vi "Abrir Archivo.vi"(11 "MulticolumnListbox in":refnum<vi>) -> (3 "Byte Stream File out":refnum<file>)   [LabVIEW 2020]
uses:
  <vilib>/Utility/miscctls.llb/LVRowAndColumnUnsignedTypeDef.ctl
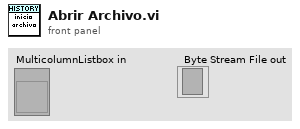
[diagram p1: front panel]
types:
  T1 = enum16{"open", "replace", "create", "open or create", "replace or create", "replace or create with confirmation"}
  T2 = typedef "LVRowAndColumnUnsignedTypeDef.ctl" = cluster{"Row":u32, "Column":u32}
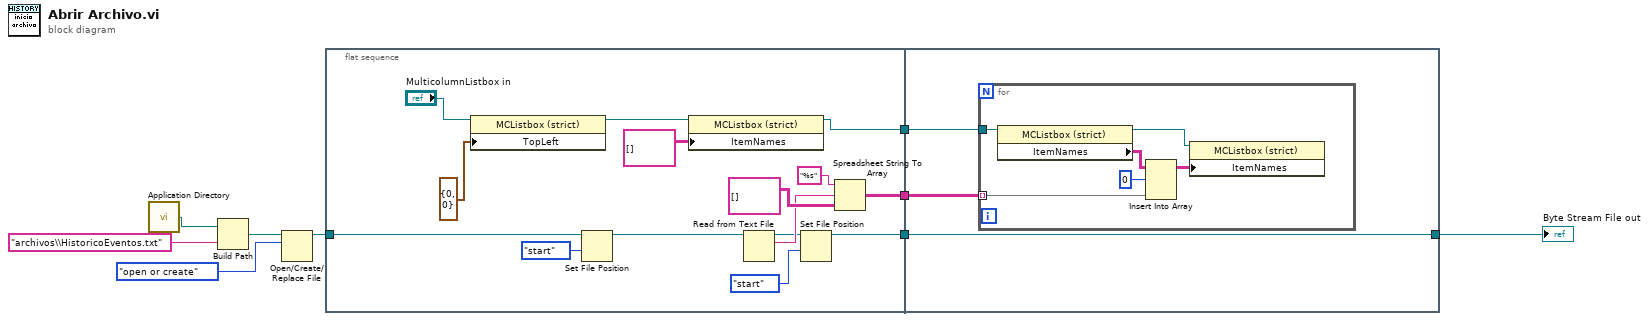
[diagram p0: block diagram]
diagram:
  n1 = call <vilib>:"Application Directory.vi"() -> ("Application Directory"=w2:path)
  n2 = Build Path(base path=w2, name or relative path="archivos\\HistoricoEventos.txt") -> (appended path=w4:path)
  n3 = Open/Create/Replace File(file path (use dialog)=w4, operation (0:open)=T1."open or create") -> (refnum out=w6:refnum<file>)  [unwired: 4 in, 2 out]
  n4 = flat-sequence {
    tunnel: w6 -> [w16]
    tunnel: [w20] -> w9
    tunnel: [w14] -> w8
    tunnel: [w13] -> w7
    tunnel: w9 -> [w27]
    tunnel: [w26] -> w1
    tunnel: w8 -> [w26]
    tunnel: w7 -> [w25]
    frame #0 {
      n5 = property on="Property Node" class="MCListbox (strict)"(reference="MulticolumnListbox in", "TopLeft"=T2 {"Row"=0, "Column"=0} ("Top Left Visible Cell")) -> (reference out=w10:refnum<vi>)  [unwired: 1 in, 1 out]
      n6 = Set File Position(refnum=w16, from (0:start)=enum16{"start", "end", "current"}."start") -> (refnum out=w15:refnum<file>)  [unwired: 2 in, 1 out]
      n7 = property on="Property Node" class="MCListbox (strict)"(reference=w10, "ItemNames"=string[][] [] ("Array")) -> (reference out=w13:refnum<vi>)  [unwired: 1 in, 1 out]
      n8 = Read from Text File(file (use dialog)=w15) -> (refnum out=w19:refnum<file>, text=w22:string)  [unwired: 2 in, 3 out]
      n9 = Set File Position(refnum=w19, from (0:start)=enum16{"start", "end", "current"}."start") -> (refnum out=w14:refnum<file>)  [unwired: 2 in, 1 out]
      n10 = Spreadsheet String To Array(format string="%s", spreadsheet string=w22, array type (2D Dbl)=string[][] [] ("Array")) -> (array=w20:string[][])  [unwired: 1 in]
    }
    frame #1 {
      n11 = for {
        tunnel: w27 -> [w31] mode=indexing
        tunnel: w25 -> [w28]
        n12 = property on="Property Node" class="MCListbox (strict)"(reference=w28) -> (reference out=w29:refnum<vi>, "ItemNames"=w33:string[][])  [unwired: 1 in, 1 out]
        n13 = Insert Into Array(array=w33, index (row)=0, new element=w31) -> (w32:string[][])  [unwired: 1 in]
        n14 = property on="Property Node" class="MCListbox (strict)"(reference=w29, "ItemNames"=w32) -> ()  [unwired: 1 in, 2 out]
      }
    }
  }
  "Byte Stream File out" <- w1
